vi "TLMythCoil.vi"(0 "String Array":string[](array[string]), 1 "Boolean input Array":dbl[](array[numeric])) -> ()   [LabVIEW 2018]
uses:
  <vilib>/Analysis/1siggen.llb/Ramp Pattern by Samples.vi
  <vilib>/DAQmx/write.llb/DAQmx Write (Analog 1D DBL 1Chan NSamp).vi
  <vilib>/DAQmx/create/channels.llb/DAQmx Create Channel (AO-Voltage-Basic).vi
  <vilib>/DAQmx/configure/timing.llb/DAQmx Timing (Sample Clock).vi
  <vilib>/DAQmx/miscellaneous.llb/DAQmx Fill In Error Info.vi
  <vilib>/Analysis/NI_AALBase.lvlib
panel:
  out "Time(s)":dbl
  out "Extr. Coil file position":i32=4
  out "End value":dbl
  out "Start Value":dbl
  out "# Coils":i32=5
  out "Device names":string[](array[string])=["Dev1/ao3", "Dev1/ao4", "Dev1/ao6", "Dev1/ao7", "Dev1/ao0"]
  out "Set Values":dbl[](array[numeric])
  out "Enable TL?":bool
  in  "rate (S/s)":dbl=1000.0 format="%0.2f"
  in  "samples":i32=100
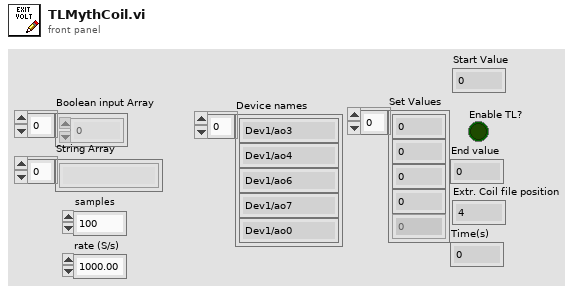
[diagram p1: front panel]
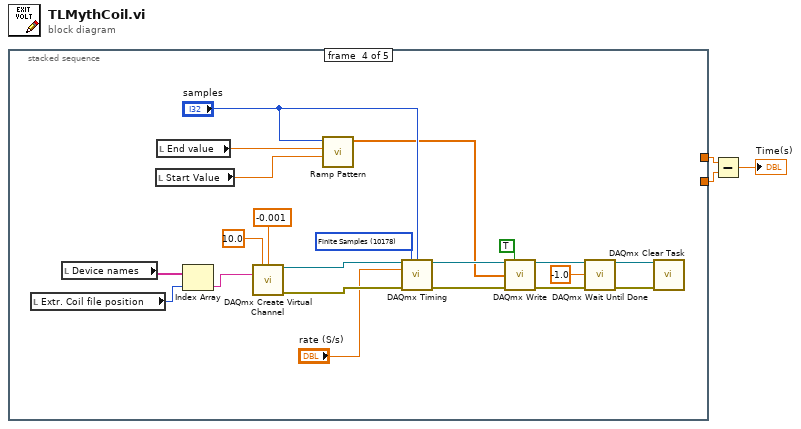
[diagram p0: block diagram]
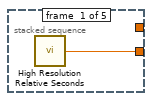
[diagram p2: hidden frame]
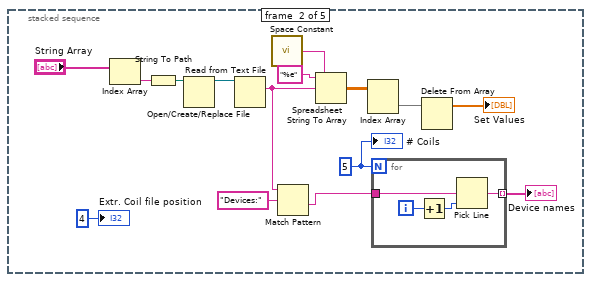
[diagram p3: hidden frame]
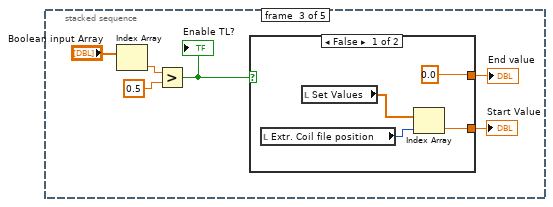
[diagram p4: hidden frame]
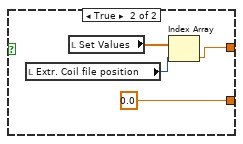
[diagram p5: hidden frame]
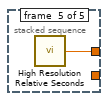
[diagram p6: hidden frame]
diagram:
  n1 = stacked-sequence {
    tunnel: [w4 _ _ _ _] -> w2
    tunnel: [_ _ _ _ w59] -> w3
    frame #0 {
      n2 = call <vilib>:"High Resolution Relative Seconds.vi"() -> ("relative seconds"=w4:dbl)
    }
    frame #1 {
      w11 = 5
      n3 = Index Array(array="String Array") -> (element=w18:string)  [unwired: 1 in]
      n4 = String To Path(string=w18) -> (path=w6:path)
      n5 = Open/Create/Replace File(file path (use dialog)=w6) -> (refnum out=w8:refnum<file>)  [unwired: 5 in, 2 out]
      n6 = Read from Text File(file (use dialog)=w8) -> (text=w14:string)  [unwired: 3 in, 3 out]
      n7 = call <vilib>:"Space Constant.vi"() -> ("String"=w16:string)
      n8 = Match Pattern(string=w14, regular expression="Devices:") -> (after substring=w12:string)  [unwired: 1 in, 3 out]
      n9 = Spreadsheet String To Array(delimiter (Tab)=w16, format string="%e", spreadsheet string=w14) -> (array=w15:dbl[][])  [unwired: 1 in]
      n10 = Index Array(array=w15) -> (element=w9:dbl[])  [unwired: 2 in]
      n11 = for {
        N: w11 -> [_]
        tunnel: w12 -> [w21]
        tunnel: [w20] -> w10 mode=indexing
        i -> [w23]
        n12 = Increment(x=w23) -> (x+1=w22:i32)
        n13 = Pick Line(multi-line string=w21, line index=w22) -> (output string=w20:string)  [unwired: 1 in]
      }
      "Device names" <- w10
      n14 = Delete From Array(array=w9) -> (array with subset deleted=→"Set Values":dbl[])  [unwired: 2 in, 1 out]
      "# Coils" <- w11
      "Extr. Coil file position" <- 4
    }
    frame #2 {
      n15 = Index Array(array="Boolean input Array") -> (element=w28:dbl)  [unwired: 1 in]
      n16 = Greater?(x=w28, y=0.5) -> (0:w26:bool)
      "Enable TL?" <- w26
      n17 = case shown="False" w26 {
        tunnel: [w31 0.0] -> w25
        tunnel: [0.0 w35] -> w24
        frame False {
          n18 = local read "Extr. Coil file position"() -> (w30:i32)
          n19 = local read "Set Values"() -> (w32:dbl[])
          n20 = Index Array(array=w32, index=w30) -> (element=w31:dbl)
        }
        frame True {
          n21 = local read "Extr. Coil file position"() -> (w34:i32)
          n22 = local read "Set Values"() -> (w36:dbl[])
          n23 = Index Array(array=w36, index=w34) -> (element=w35:dbl)
        }
      }
      "Start Value" <- w25
      "End value" <- w24
    }
    frame #3 {
      w45 = 10178 items=["Finite Samples"=10178, "Continuous Samples"=10123, "Hardware Timed Single Point"=12522] ("sample mode")
      n24 = local read "Extr. Coil file position"() -> (w38:i32)
      n25 = local read "Device names"() -> (w41:string[])
      n26 = local read "Start Value"() -> (w43:dbl)
      n27 = local read "End value"() -> (w44:dbl)
      n28 = Index Array(array=w41, index=w38) -> (element=w40:string)
      n29 = call-poly <vilib>:"DAQmx Create Virtual Channel.vi"("maximum value"=10.0, "minimum value"=-0.001, "physical channels"=w40) -> ("task out"=w54:refnum<k21>, "error out"=w55:errorcluster)  [unwired: 11 in]
      n30 = call-poly <vilib>:"Ramp Pattern.vi"("start"=w43, "end"=w44, "samples"="samples") -> ("Ramp Pattern"=w39:dbl[])  [unwired: 7 in, 1 out]
      n31 = call-poly <vilib>:"DAQmx Timing.vi"("task/channels in"=w54, "sample mode"=w45, "samples per channel"="samples", "rate"="rate (S/s)", "error in"=w55) -> ("task out"=w57:refnum<k21>, "error out"=w56:errorcluster)  [unwired: 9 in]
      n32 = call-poly <vilib>:"DAQmx Write.vi"("task/channels in"=w57, "auto start"=TRUE, "data"=w39, "error in"=w56) -> ("task out"=w53:refnum<k21>, "error out"=w52:errorcluster)  [unwired: 9 in, 1 out]
      n33 = call <vilib>:"DAQmx Wait Until Done.vi"("task/channels in"=w53, "timeout (sec)"=-1.0, "error in"=w52) -> ("task out"=w51:refnum<k21>, "error out"=w50:errorcluster)  [unwired: 11 in]
      n34 = call <vilib>:"DAQmx Clear Task.vi"("task in"=w51, "error in"=w50) -> ()  [unwired: 13 in, 1 out]
    }
    frame #4 {
      n35 = call <vilib>:"High Resolution Relative Seconds.vi"() -> ("relative seconds"=w59:dbl)
    }
  }
  n36 = Subtract(x=w3, y=w2) -> (x-y=→"Time(s)":dbl)
